vi "ReadRadsensoren.vi"(8 "error in (no error)":errorcluster, 9 "milliseconds to wait":u32, 10 "FPGA VI Reference Out":refnum<k20>) -> (0 "error out":errorcluster)   [LabVIEW 2016]
uses:
  <vilib>/Utility/error.llb/Error Cluster From Error Code.vi
  <vilib>/rvi/errors/niLvFpgaAdjustHostInterfaceError.vi
  Globale Variablen VI/RadSensoren.vi
  <vilib>/rvi/interface/nirviReadWriteControl/nirviReadWriteControl.xnode
  NiFpgaLv.dll
  <vilib>/rvi/interface/Simulation/niFpgaSimulationCallBeginRW.vi
panel:
  out "vHR":sgl
  out "vHL":sgl
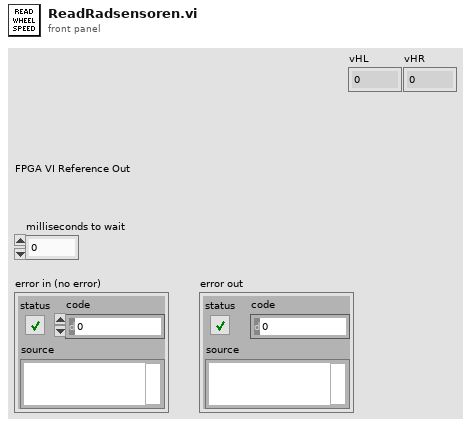
[diagram p1: front panel]
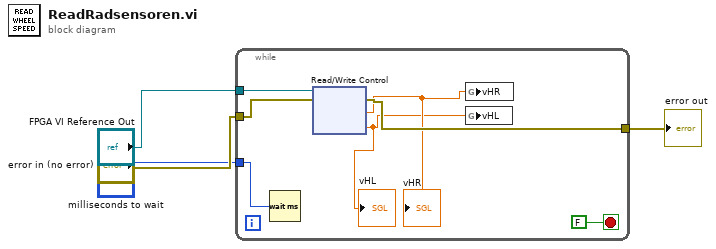
[diagram p0: block diagram]
diagram:
  n1 = while {
    tunnel: "error in (no error)" -> [w8]
    tunnel: [w7] -> w4
    tunnel: "milliseconds to wait" -> [w10]
    tunnel: "FPGA VI Reference Out" -> [w9]
    stop <- FALSE stop-if-true
    n2 = Wait (ms)(milliseconds to wait=w10) -> ()  [unwired: 1 out]
    n3 = xnode "Read/Write Control"("FPGA VI Reference In"=w9, "error in"=w8) -> ("error out"=w7:errorcluster, "vHR"=w6:sgl, "vHL"=w5:sgl)  [unwired: 1 out]
    "vHL" <- w5
    "vHR" <- w6
    n4 = global write "RadSensoren.vi" "vHR"(w6) -> ()
    n5 = global write "RadSensoren.vi" "vHL"(w5) -> ()
  }
  "error out" <- w4
